vi "Functional Imaging-Return ROI Z-plane.vi"(9 "ROI index (zero based)":i32, 11 "Functional Parameters":T1) -> (3 "Zero-based index of the Z-plane the indexed ROI belongs to":i32)   [LabVIEW 2017]
uses:
  Typedefs/Functional Parameters Cluster.ctl
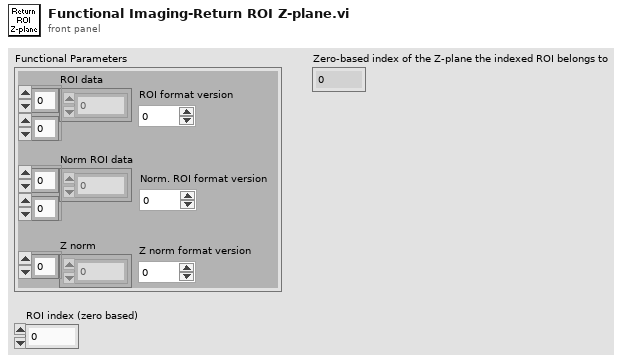
[diagram p1: front panel]
types:
  T1 = typedef "Functional Parameters Cluster.ctl" = cluster{"ROI data":dbl[][], "ROI format version":i32, "Norm ROI data":dbl[][], "Norm. ROI format version":i32, "Z norm":dbl[], "Z norm format version":i32}
  T2 = typedef "ROI file columns mapping.ctl" = cluster{"\"ROI index\" column index":i32, "\"ROI ID\" column index":i32, "\"ROI Time (ns)\" column index":i32, "\"Pixels in ROI\" column index":i32, "\"X (X start)\" column index":i32, "\"Y (Y start)\" column index":i32, "\"Z (Z start)\" column index":i32, "\"X (X stop)\" column index":i32, "\"Y (Y stop)\" column index":i32, "\"Z (Z stop)\" column index":i32, "\"Angle (deg)\" column index":i32, "Composite ID":i32, "Number of lines":i32, "Frame Size":i32, "Zoom":i32, "Laser Power (%)":i32, "ROI group ID":i32}
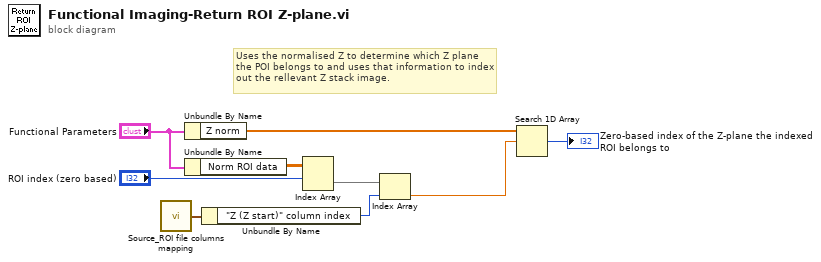
[diagram p0: block diagram]
diagram:
  # "Uses the normalised Z to determine which Z plane the POI belongs to and uses that information to index out the rellevant Z stack image."
  n1 = call "Source_ROI file columns mapping.vi"() -> ("ROI file columns mapping"=w4:T2)  [unwired: 1 in]
  n2 = Unbundle By Name("Functional Parameters") -> ("Z norm"=w8:dbl[])
  n3 = Unbundle By Name("Functional Parameters") -> ("Norm ROI data"=w2:dbl[][])
  n4 = Unbundle By Name(w4) -> ("\"Z (Z start)\" column index"=w5:i32)
  n5 = Index Array(array=w2, index (row)="ROI index (zero based)") -> (element=w1:dbl[])  [unwired: 1 in]
  n6 = Index Array(array=w1, index=w5) -> (element=w9:dbl)
  n7 = Search 1D Array(1D array=w8, element=w9) -> (index of element=→"Zero-based index of the Z-plane the indexed ROI belongs to":i32)  [unwired: 1 in]
